vi "Ophir PyroPower.vi"(0 "Visa Session":refnum<visa-resource-name>, 1 "error in (no error)":errorcluster) -> (2 "dup Visa Session":refnum<visa-resource-name>, 3 "Value Number":dbl format="%.3e", 4 "Value String":string, 5 "error out":errorcluster)   [LabVIEW 2017]
doc: "PyroPower.vi returns power measurement from instrument with PyroElectric and NanoJoule-Meter head.\nVersion 1.00\nLast Updated 16 March 2005\n\nThis VI doesn't include the Power Configuration Initialization\nof the Device.\n\nInputs:\nVisa Session\nErrorIn\n\nOutputs:\ndup Visa Session\nValue Number is the Measurement Value\nValue String is the Measurement String\nNote:\nIn case of Overrange Measure The string contains *OVER\nErrorOut\nReturns Error n# -1339 when Measurement Failed"
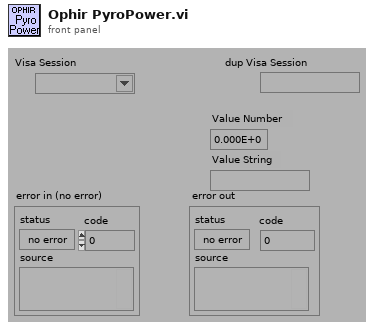
[diagram p1: front panel]
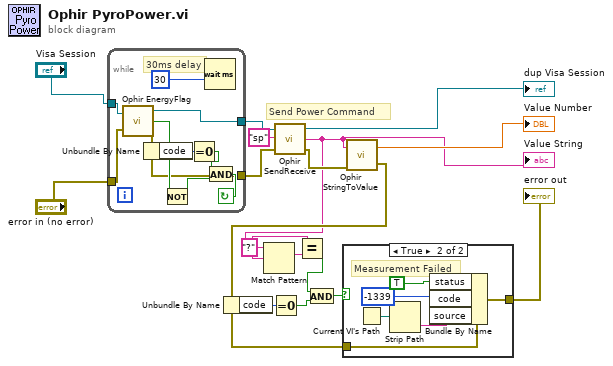
[diagram p0: block diagram]
diagram:
  w7 = "?"
  # "Send Power Command"
  n1 = while {
    tunnel: [w20] -> w14
    tunnel: "error in (no error)" -> [w24]
    tunnel: [w25] -> w13
    tunnel: "Visa Session" -> [w26]
    stop <- w23 continue-if-true
    # "30ms delay"
    n2 = call "Ophir EnergyFlag.vi"("Visa Session"=w26, "error in (no error)"=w24) -> ("dup Visa Session"=w25:refnum<visa-resource-name>, "Energy Flag?"=w27:bool, "error out"=w20:errorcluster)
    n3 = Unbundle By Name(w20) -> ("code"=w21:i32)
    n4 = Not(x=w27) -> (.not. x?=w22:bool)
    n5 = Equal To 0?(x=w21) -> (x = 0?=w19:bool)
    n6 = Wait (ms)(milliseconds to wait=30) -> ()  [unwired: 1 out]
    n7 = And(x=w19, y=w22) -> (x .and. y?=w23:bool)
  }
  n8 = call "Ophir SendReceive.vi"("error in (no error)"=w14, "Command"="sp", "Visa Session"=w13) -> ("error out"=w12:errorcluster, "Frame Output"=w2:string, "dup Visa Session"=→"dup Visa Session":refnum<visa-resource-name>)
  "Value String" <- w2
  n9 = Match Pattern(string=w2, regular expression=w7) -> (match substring=w6:string)  [unwired: 4 out]
  n10 = Equal?(x=w7, y=w6) -> (x = y?=w5:bool)
  n11 = call "Ophir StringToValue.vi"("error in (no error)"=w12, "Frame"=w2) -> ("error out"=w3:errorcluster, "Value"=→"Value Number":dbl)
  n12 = Unbundle By Name(w3) -> ("code"=w9:i32)
  n13 = Equal To 0?(x=w9) -> (x = 0?=w8:bool)
  n14 = And(x=w5, y=w8) -> (x .and. y?=w4:bool)
  n15 = case shown="True" w4 {
    tunnel: w3 -> [w28 w31]
    tunnel: [w28 w30] -> w1
    frame False {
      # "No Error or \nError already exists"
    }
    frame True {
      # "Measurement Failed"
      n16 = Current VI's Path() -> (path=w29:path)
      n17 = Strip Path(path=w29) -> (name=w32:string)  [unwired: 1 out]
      n18 = Bundle By Name(cluster=w31, "status"=TRUE, "code"=-1339, "source"=w32) -> (w30:errorcluster)
    }
  }
  "error out" <- w1
